vi "Initialize From Settings.vi"(8 "error in":errorcluster, 10 "settings":cluster{"key":string, "value":string}[](array[cluster]), 11 "RDMA Tx Transfer Configuration in":refnum<class "RDMA Transfer Tx Configuration.lvclass">) -> (0 "error out":errorcluster, 3 "RDMA Tx Transfer Configuration out":refnum<class "RDMA Transfer Tx Configuration.lvclass">)   [LabVIEW 2020, in "RDMA.lvlib" / "RDMA Transfer Tx Configuration.lvclass"]
uses:
  RDMA Transfer Tx Configuration.lvclass
  Tx Transfer Settings.ctl
  RDMA Transfer Tx Configuration.lvclass/RDMA Transfer Tx Configuration.ctl
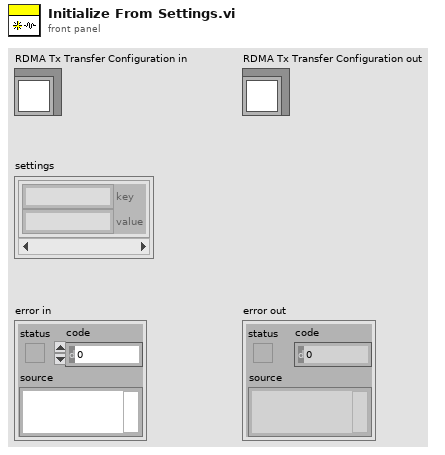
[diagram p1: front panel]
types:
  T1 = typedef "RDMA.lvlib/RDMA Transfer Tx Configuration.lvclass/Tx Transfer Settings.ctl" = cluster{"local address":u32, "local port":u16, "destination address":u32, "destination port":u16, "decimation":u16}
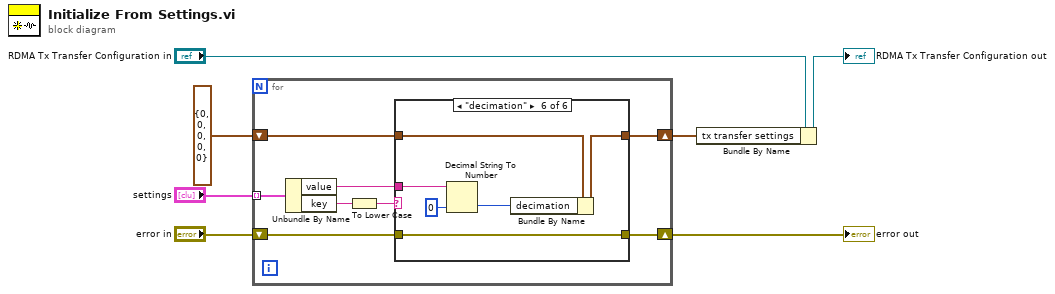
[diagram p0: block diagram]
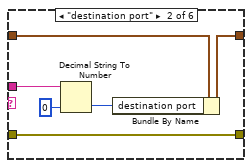
[diagram p3: hidden frame]
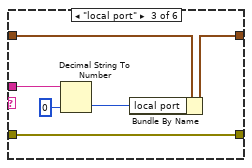
[diagram p4: hidden frame]
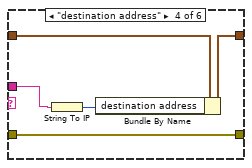
[diagram p5: hidden frame]
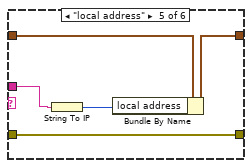
[diagram p6: hidden frame]
diagram:
  n1 = for {
    shift-right: [w11] -> w1
    shift-left: "error in" -> [w15]
    shift-right: [w13] -> w5
    shift-left: T1 {"local address"=0, "local port"=0, "destination address"=0, "destination port"=0, "decimation"=0} ("tx transfer settings") -> [w14]
    tunnel: "settings" -> [w10] mode=indexing
    n2 = Unbundle By Name(w10) -> ("value"=w8:string, "key"=w9:string)
    n3 = To Lower Case(string=w9) -> (all lower case string=w12:string)
    n4 = case shown="\"decimation\"" w12 {
      tunnel: w15 -> [w16 w21 w27 w32 w37 w43]
      tunnel: w8 -> [_ w20 w26 w31 w36 w42]
      tunnel: w14 -> [w17 w23 w29 w34 w39 w45]
      tunnel: [w17 w22 w28 w33 w38 w44] -> w13
      tunnel: [w16 w21 w27 w32 w37 w43] -> w11
      frame Default {
        # "Unknown Setting."
      }
      frame "destination port" {
        n5 = Decimal String To Number(string=w20, default (0L)=u16 0 ("default (0 I32)")) -> (number=w19:u16)  [unwired: 1 in, 1 out]
        n6 = Bundle By Name(cluster=w23, "destination port"=w19) -> (w22:T1)
      }
      frame "local port" {
        n7 = Decimal String To Number(string=w26, default (0L)=u16 0 ("default (0 I32)")) -> (number=w25:u16)  [unwired: 1 in, 1 out]
        n8 = Bundle By Name(cluster=w29, "local port"=w25) -> (w28:T1)
      }
      frame "destination address" {
        n9 = String To IP(1:w31) -> (0:w30:u32)
        n10 = Bundle By Name(cluster=w34, "destination address"=w30) -> (w33:T1)
      }
      frame "local address" {
        n11 = String To IP(1:w36) -> (0:w35:u32)
        n12 = Bundle By Name(cluster=w39, "local address"=w35) -> (w38:T1)
      }
      frame "decimation" {
        n13 = Decimal String To Number(string=w42, default (0L)=u16 0 ("default (0 I32)")) -> (number=w41:u16)  [unwired: 1 in, 1 out]
        n14 = Bundle By Name(cluster=w45, "decimation"=w41) -> (w44:T1)
      }
    }
  }
  "error out" <- w1
  n15 = Bundle By Name(cluster="RDMA Tx Transfer Configuration in", "tx transfer settings"=w5) -> (→"RDMA Tx Transfer Configuration out":refnum<class "RDMA Transfer Tx Configuration.lvclass">)
